vi "is a.vi"(8 "error in (no error)":errorcluster, 11 "CCD in":refnum<class "Inclinometer.lvclass">) -> (0 "error out":errorcluster, 2 "is a":string, 3 "CCD out":refnum<class "Inclinometer.lvclass">)   [LabVIEW 2016, in "Hardware.lvlib" / "Inclinometer.lvlib" / "Inclinometer.lvclass"]
uses:
  <userlib>/Common Components/Hardware/Inclinometer/Inclinometer/Inclinometer.lvclass
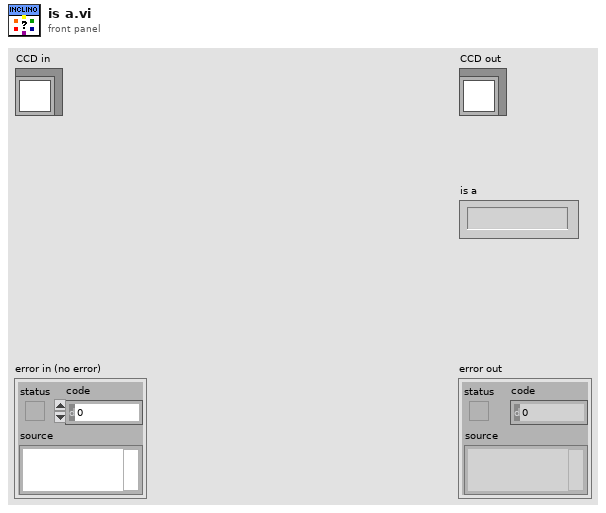
[diagram p1: front panel]
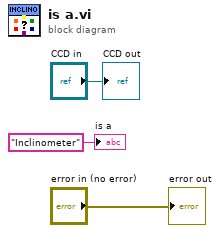
[diagram p0: block diagram]
diagram:
  "error out" <- "error in (no error)"
  "CCD out" <- "CCD in"
  "is a" <- "Inclinometer" ("is a")
